vi "GetStep.vi"(9 "Child (Step)":string, 10 "Parent (Script)":string, 11 "Scripts":T1[](array[typedef])) -> (1 "Step":i32, 2 "Script":i32, 3 "Step Found":bool)   [LabVIEW 2024, in "Setting_Screen.lvlib"]
uses:
  Setting_Screen.lvlib
  ScriptDetails.ctl
  CurrentStep.ctl
  StepType.ctl
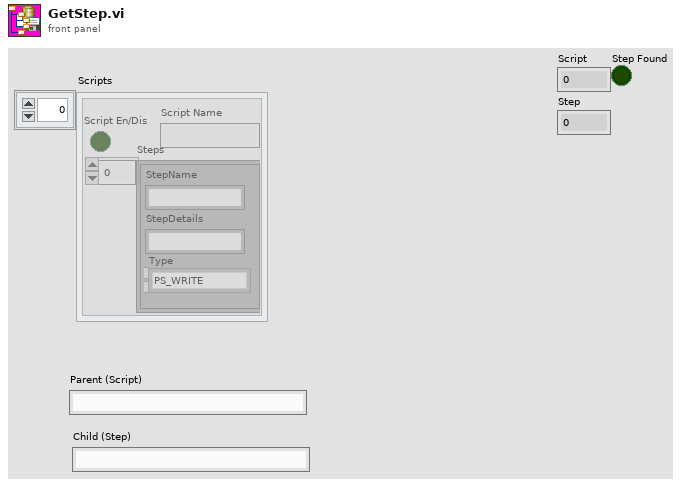
[diagram p1: front panel]
types:
  T1 = typedef "Setting_Screen.lvlib/ScriptDetails.ctl" = cluster{"Script Name":string, "Steps":T2[], "Script En/Dis":bool}
  T2 = typedef "Setting_Screen.lvlib/CurrentStep.ctl" = cluster{"StepName":string, "StepDetails":string, "Type":T3}
  T3 = typedef "Setting_Screen.lvlib/StepType.ctl" = enum16{"RELAY_CHANNEL_WRITE", "PS_WRITE", "READ_DATA", "DMM_CONFIG", "DAQ_CONFIG", "PCAN_Read", "PCAN_Write", "Camera", "MCU_Flashing", "Noeway_Flashing", "SSL_Certification"}
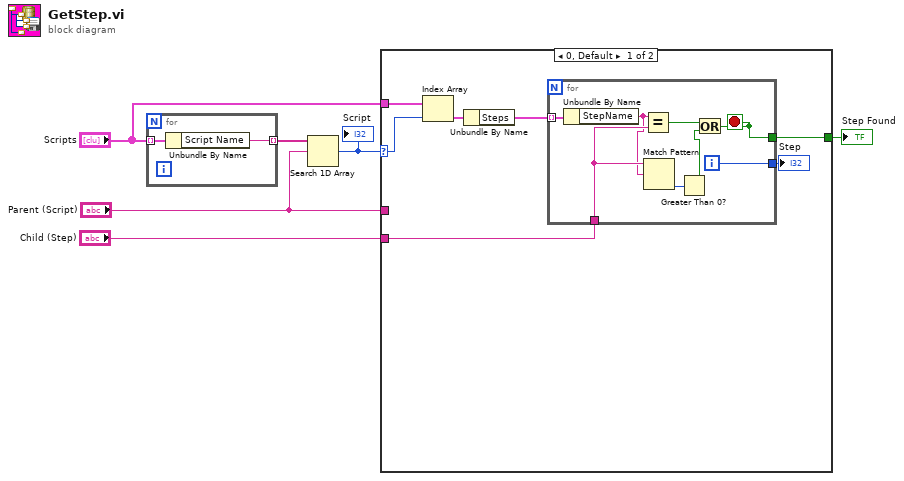
[diagram p0: block diagram]
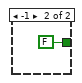
[diagram p2: hidden frame]
diagram:
  n1 = for {
    tunnel: "Scripts" -> [w8] mode=indexing
    tunnel: [w7] -> w6 mode=indexing
    n2 = Unbundle By Name(w8) -> ("Script Name"=w7:string)
  }
  n3 = Search 1D Array(1D array=w6, element="Parent (Script)") -> (index of element=w5:i32)  [unwired: 1 in]
  "Script" <- w5
  n4 = case shown="0, Default" w5 {
    selector: w5 -> [w14 _]
    tunnel: "Child (Step)" -> [w11 _]
    tunnel: "Parent (Script)" -> [_ _]
    tunnel: "Scripts" -> [w15 _]
    tunnel: [w9 FALSE] -> w1
    frame 0, Default {
      n5 = Index Array(array=w15, index=w14) -> (element=w13:T1)
      n6 = Unbundle By Name(w13) -> ("Steps"=w12:T2[])
      n7 = for {
        tunnel: w12 -> [w23] mode=indexing
        tunnel: w11 -> [w19]
        tunnel: [w22] -> w10
        tunnel: [w20] -> w9
        i -> [w22]
        stop <- w20 stop-if-true
        n8 = Unbundle By Name(w23) -> ("StepName"=w18:string)
        n9 = Equal?(x=w18, y=w19) -> (x = y?=w21:bool)
        n10 = Match Pattern(string=w19, regular expression=w18) -> (offset past match=w17:i32)  [unwired: 1 in, 3 out]
        n11 = Greater Than 0?(x=w17) -> (x > 0?=w16:bool)
        n12 = Or(x=w21, y=w16) -> (x .or. y?=w20:bool)
      }
      "Step" <- w10
    }
    frame -1 {
    }
  }
  "Step Found" <- w1
